vi "Snap Camera Image.vi"(7 "Test Recipe in":refnum<class "Test Recipe.lvclass">, 10 "Camera":refnum<class "Camera.lvclass">, 11 "Path":path) -> (0 "error out":errorcluster, 2 "Color Artifacts Found":bool, 3 "LEDs Found":u32)   [LabVIEW 2015]
uses:
  Classes/Instruments/Camera/Camera/Class/Camera.lvclass
  Classes/Test Recipe/Class/Test Recipe.lvclass
  Classes/Instruments/Camera/Camera/Vision Algorithm/Count LEDS on Image/Count LEDs on Image.lvclass
  Classes/Instruments/Camera/Camera/Vision Algorithm/Find Color Artifacts/Find Color Artifacts.lvclass
  Classes/Instruments/Camera/Camera/Vision Algorithm/Find Color Artifacts/Find Color Artifacts.lvclass/Find Color Artifacts.ctl
  Classes/Instruments/Camera/Camera/Vision Algorithm/Count LEDS on Image/Count LEDs on Image.lvclass/Count LEDs on Image.ctl
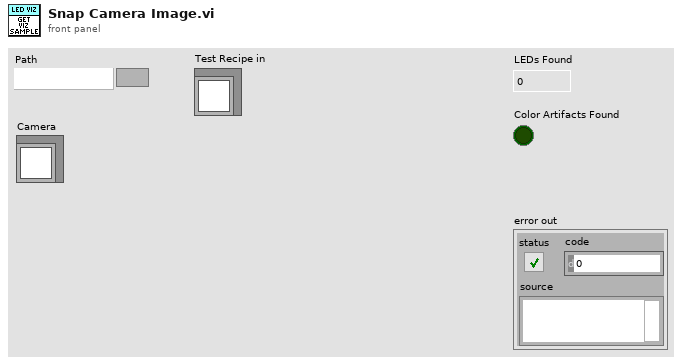
[diagram p1: front panel]
types:
  T1 = cluster{"Red Range":cluster{"Lower value":i32, "Upper value":i32}, "Green Range":cluster{"Lower value":i32, "Upper value":i32}, "Blue Range":cluster{"Lower value":i32, "Upper value":i32}}
  T2 = typedef "IMAQ Rectangle" = cluster{"Left":i32, "Top":i32, "Right":i32, "Bottom":i32, "Rotation":dbl}
  T3 = cluster{"Threshold":u32, "Min Size":u32, "Max Size":u32, "Use Max Size":bool}
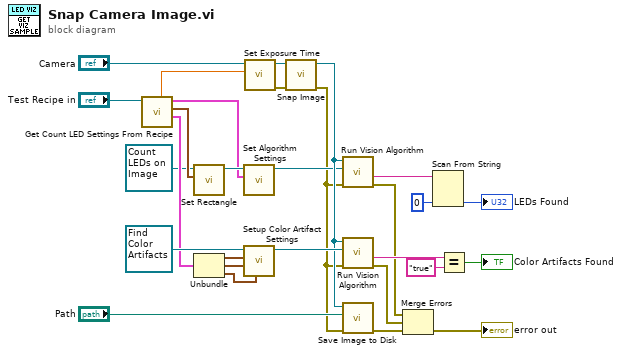
[diagram p0: block diagram]
diagram:
  n1 = call "Get Count LED Settings From Recipe.vi"("Test Recipe in"="Test Recipe in") -> ("Threshold Values"=w20:T1, "Rectangle"=w23:T2, "Search Settings"=w7:T3, "Exposure Speed"=w10:dbl)  [unwired: 6 in, 1 out]
  n2 = call "Set Rectangle.vi"("Rectangle"=w23, "Count LEDs on Image in"=refnum<class "Count LEDs on Image.lvclass"> refnum ("Camera.lvlib:Count LEDs on Image.lvclass")) -> ("Count LEDs on Image out"=w9:refnum<class "Count LEDs on Image.lvclass">)  [unwired: 8 in, 1 out]
  n3 = Unbundle(w20) -> ("Red Range"=w19:cluster{"Lower value":i32, "Upper value":i32}, "Green Range"=w18:cluster{"Lower value":i32, "Upper value":i32}, "Blue Range"=w17:cluster{"Lower value":i32, "Upper value":i32})
  n4 = call "Set Algorithm Settings.vi"("Search Settings"=w7, "Count LEDs on Image in"=w9) -> ("Count LEDs on Image out"=w6:refnum<class "Count LEDs on Image.lvclass">)  [unwired: 8 in, 1 out]
  n5 = call "Setup Color Artifact Settings.vi"("Blue Range"=w17, "Green Range"=w18, "Red Range"=w19, "Find Color Artifacts in"=refnum<class "Find Color Artifacts.lvclass"> refnum ("Camera.lvlib:Find Color Artifacts.lvclass")) -> ("Find Color Artifacts out"=w16:refnum<class "Find Color Artifacts.lvclass">)  [unwired: 6 in, 1 out]
  n6 = call-dynamic "Set Exposure Time.vi"("Exposure Time"=w10, "Acrobat Template in"="Camera") -> ("error out"=w14:errorcluster, "Acrobat Template out"=w27:refnum<class "Camera.lvclass">)  [unwired: 8 in]
  n7 = call-dynamic "Snap Image.vi"("error in (no error)"=w14, "Acrobat Template in"=w27) -> ("error out"=w1:errorcluster, "Acrobat Template out"=w15:refnum<class "Camera.lvclass">)  [unwired: 8 in]
  n8 = call "Run Vision Algorithm.vi"("error in (no error)"=w1, "Vision Algorithm"=w6, "Camera in"=w15) -> ("error out"=w3:errorcluster, "Data"=w22:string)  [unwired: 4 in, 3 out]
  n9 = call "Run Vision Algorithm.vi"("error in (no error)"=w1, "Vision Algorithm"=w16, "Camera in"=w15) -> ("error out"=w2:errorcluster, "Data"=w13:string)  [unwired: 4 in, 3 out]
  n10 = call "Save Image to Disk.vi"("error in (no error)"=w1, "Path"="Path", "Camera in"=w15) -> ("error out"=w5:errorcluster)  [unwired: 8 in]
  n11 = Merge Errors(w3, w2, w5) -> (→"error out":errorcluster)
  n12 = Scan From String(input string=w22, default 1=0) -> (output 1=→"LEDs Found":i32)  [unwired: 3 in, 3 out]
  n13 = Equal?(x=w13, y="true") -> (x = y?=→"Color Artifacts Found":bool)
